vi "4-9 PiPoPa.vi"() -> ()   [LabVIEW 2014]
doc: "This VI illustrates how to acquire a finite number of samples from a specified device. It requires the use of a microphone attached to the sound card. You can specify the number of samples to acquire, sample rate, number of channels and a bit rate per sample.\n------------------------------------\nAuther: Koji Ohashi\nModified: Hirotake Watashima\nCopyright (c) 2020 Japan LabVIEW Users Group, Volunteer members.\nThis VI is released under the MIT License.\nhttp://opensource.org/licenses/mit-license.php\n------------------------------------"
uses:
  <vilib>/sound2/lvsound2.llb/Sampling Mode.ctl
  <vilib>/sound2/lvsound2.llb/Sound Data Format.ctl
  <vilib>/sound2/lvsound2.llb/Sound Output Write (DBL Single).vi
  <vilib>/sound2/lvsound2.llb/Sound Output Set Volume (Single).vi
panel:
  in  "milliseconds to wait":u32=100
  out "Low Frequency":dbl
  out "High Frequency":dbl
  out "error out":errorcluster
  in  "String":string="147*2580369#ABCD"
  in  "volume":dbl(slide)=51.02040816326531 scale=0.0..100.0
  out "Sound Output":waveform(dbl)(graph)
  in  "再生時間(sec)":dbl=0.1
  in  "device ID (Out)":u32
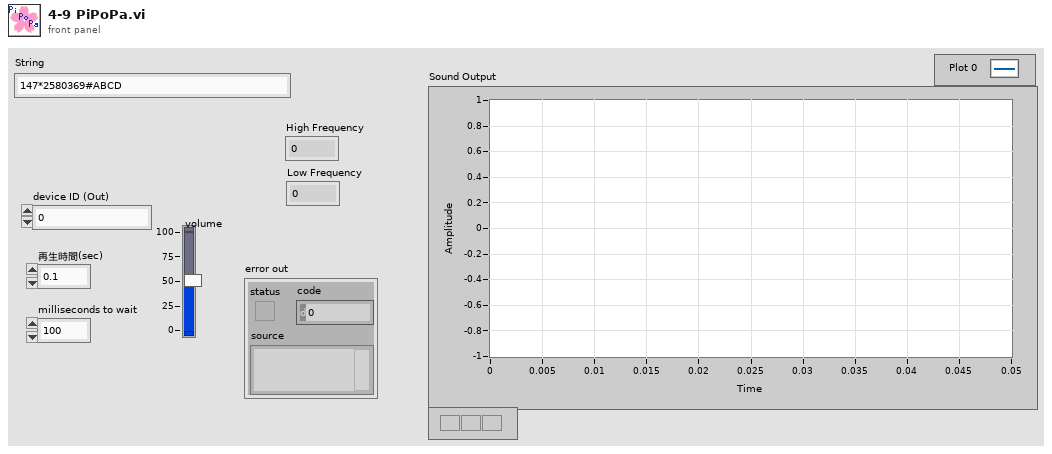
[diagram p1: front panel]
types:
  T1 = typedef "Sound Data Format.ctl" = cluster{"sample rate (S/s)":dbl, "number of channels":i32, "bits per sample":i32}
  T2 = typedef "Sampling Mode.ctl" = i32
  T3 = typedef "Sound Output Task ID.ctl" = u32
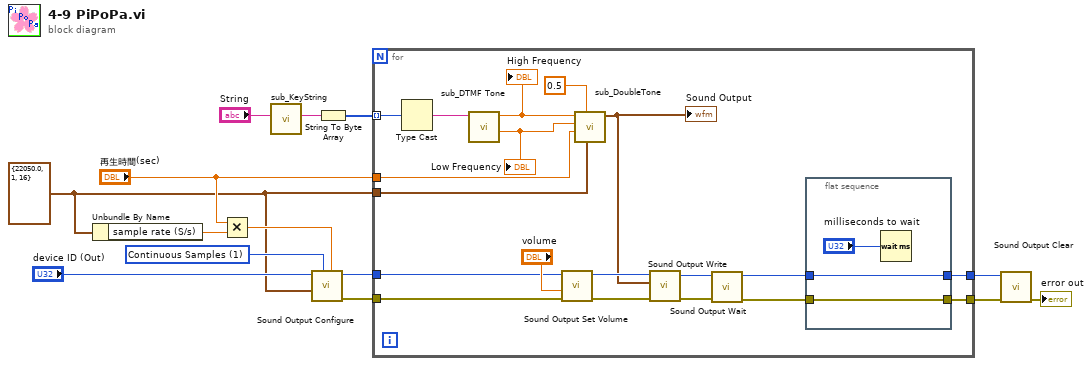
[diagram p0: block diagram]
diagram:
  w4 = T1 {"sample rate (S/s)"=22050.0, "number of channels"=1, "bits per sample"=16} ("Sound Format")
  w11 = T2 1 items=["Finite Samples", "Continuous Samples"] ("sample mode")
  n1 = Unbundle By Name(w4) -> ("sample rate (S/s)"=w7:dbl)
  n2 = Multiply(x="再生時間(sec)", y=w7) -> (x*y=w5:dbl)
  n3 = call "sub_KeyString.vi"("String"="String") -> ("Key String"=w1:string)  [unwired: 10 in]
  n4 = call <vilib>:"Sound Output Configure.vi"("number of samples/ch"=w5, "sample mode"=w11, "sound format"=w4, "device ID"="device ID (Out)") -> ("error out"=w3:errorcluster, "task ID"=w12:T3)  [unwired: 6 in]
  n5 = String To Byte Array(string=w1) -> (unsigned byte array=w14:u8[])
  n6 = for {
    tunnel: w12 -> [w21]
    tunnel: w4 -> [w23]
    tunnel: "再生時間(sec)" -> [w24]
    tunnel: w14 -> [w16] mode=indexing
    tunnel: [w22] -> w9
    tunnel: [w18] -> w10
    tunnel: w3 -> [w17]
    n7 = Type Cast(x=w16) -> (*(type *) &x=w15:string)  [unwired: 1 in]
    n8 = call "sub_DTMF Tone.vi"("Key Character"=w15) -> ("Low Frequency"=w27:dbl, "High Frequency"=w28:dbl)  [unwired: 8 in, 1 out]
    "High Frequency" <- w28
    "Low Frequency" <- w27
    n9 = call-poly <vilib>:"Sound Output Set Volume.vi"("error in (no error)"=w17, "volume"="volume", "task ID"=w21) -> ("error out"=w30:errorcluster, "task ID out"=w31:T3)  [unwired: 7 in]
    n10 = call "sub_DoubleTone.vi"("Sound Format"=w23, "amplitude"=0.5, "Play time (sec)"=w24, "2nd frequency (Hz)"=w27, "1st frequency (Hz)"=w28) -> ("signal out"=w25:waveform(dbl))  [unwired: 4 in, 2 out]
    "Sound Output" <- w25
    n11 = call-poly <vilib>:"Sound Output Write.vi"("error in (no error)"=w30, "data"=w25, "task ID"=w31) -> ("error out"=w33:errorcluster, "task ID out"=w32:T3)  [unwired: 7 in]
    n12 = call <vilib>:"Sound Output Wait.vi"("error in (no error)"=w33, "task ID"=w32) -> ("error out"=w20:errorcluster, "task ID out"=w19:T3)  [unwired: 8 in]
    n13 = flat-sequence {
      tunnel: [w36] -> w22
      tunnel: w20 -> [w36]
      tunnel: [w34] -> w18
      tunnel: w19 -> [w34]
      frame #0 {
        n14 = Wait (ms)(milliseconds to wait="milliseconds to wait") -> ()  [unwired: 1 out]
      }
    }
  }
  n15 = call <vilib>:"Sound Output Clear.vi"("error in (no error)"=w9, "task ID"=w10) -> ("error out"=→"error out":errorcluster)  [unwired: 9 in]
